vi "sort2darrayby1stcolumt.vi"(8 "array":i32[](array[numeric]), 11 "we array":i32[](array[numeric])) -> (2 "Array":i32[][](array[numeric]))   [LabVIEW 2013]
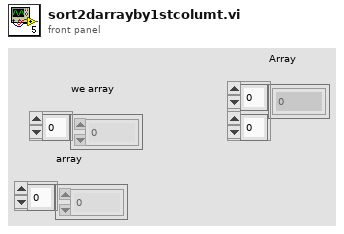
[diagram p1: front panel]
types:
  T1 = cluster{"dimension size":i32, "dimension size":i32}[]
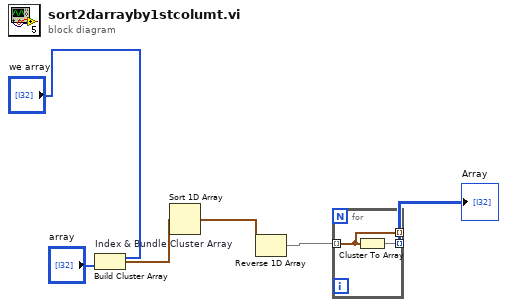
[diagram p0: block diagram]
diagram:
  n1 = Build Cluster Array "Index & Bundle Cluster Array"("we array", "array") -> (w2:T1)
  n2 = Sort 1D Array(array=w2) -> (sorted array=w3:T1)
  n3 = Reverse 1D Array(array=w3) -> (reversed array=w4:T1)
  n4 = for {
    tunnel: [w7] -> _ mode=indexing
    tunnel: [w8] -> w6 mode=indexing
    tunnel: w4 -> [w7] mode=indexing
    n5 = Cluster To Array(cluster=w7) -> (array=w8:i32[])
  }
  "Array" <- w6
